vi "GetClassInfoDialog.vi"(0 "ClassWriterRefIn":refnum<class "ClassWriterNative.lvclass">, 1 "ClassItemRefIn":refnum<vi>, 5 "error in (no error)":errorcluster) -> (14 "ClassWriterRefOut":refnum<class "ClassWriterNative.lvclass">, 19 "error out":errorcluster)   [LabVIEW 2020, in "ClassWriterNative.lvclass"]
uses:
  <resource>/Framework/Providers/Open_GDS/ClassProviders/Provider_LvNativeClass/ClassWriterNative_class/ClassWriterNative.lvclass
  <resource>/Framework/Providers/Open_GDS/ClassProviders/Common/ScriptingFunctions/Scripting_ConnectorPanePatternType.ctl
  <resource>/Framework/Providers/Open_GDS/ClassProviders/Common/LvClass_class/GDSLvClass_PlugIn.ctl
  <resource>/Framework/Providers/Open_GDS/ClassProviders/Common/LvClass_class/GDSLvClass_PlugInTypes.ctl
  Instance           1 26Saved   GetClassInfoDialog .vi
panel:
  out "Connector Pane":T1 items=["4x4x4", "5x6x5", "6x8x6"]
  in  "_SaveChanges":bool
  in  "_ClassPlugIns":T2(array[cluster]) caption="PlugIns / Design Patterns"
  in  "_EditPlugIn":bool
  in  "_OK":bool
  out "_ClassDescription":string caption="Class description"
  out "_ClassTemplateVersion":string caption="Class Template Version"
  out "_ClassTemplateUsed":string caption="Class Template Used"
  out "_ClassProviderName":string caption="Class Provider Name"
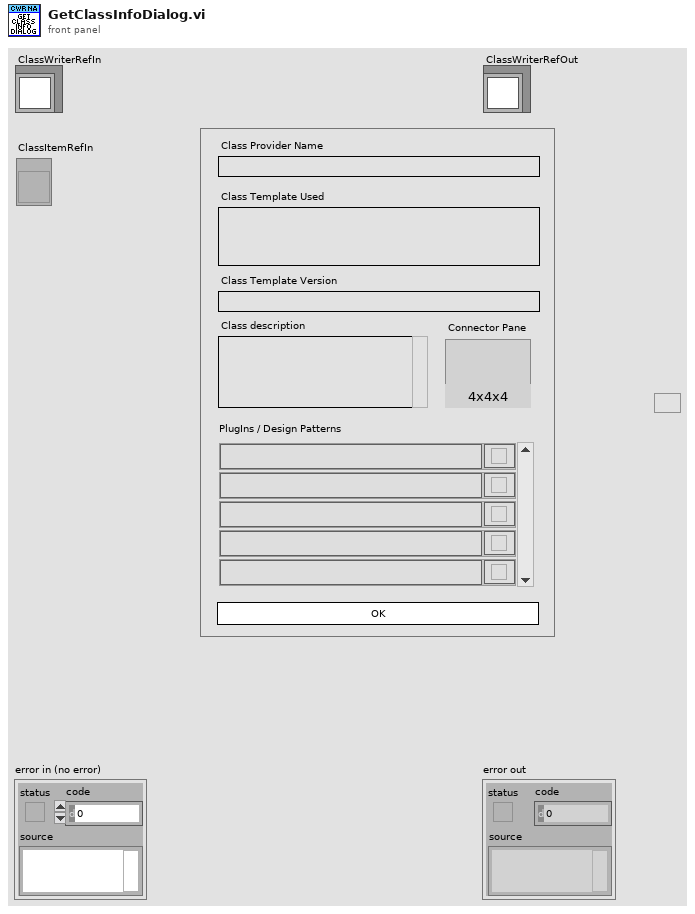
[diagram p1: front panel]
types:
  T1 = typedef "Scripting_ConnectorPanePatternType.ctl" = u16
  T2 = cluster{"_ClassPlugIn 2":string, "Remove":bool, "Block":bool}[]
  T3 = typedef "GDSLvClass_PlugIn.ctl" = cluster{"Type":T4, "ID":string, "Version":string, "Path":path, "Name":string, "Data":variant}
  T4 = typedef "GDSLvClass_PlugInTypes.ctl" = enum16{"DesignPattern", "MethodTypes"}
  T5 = cluster{"_ClassPlugIn 2":string, "_RemovePlugIn":bool, "Block":bool}
  T6 = typedef "GDSLvCLass_ClassSettingsType.ctl" = cluster{"ClassProviderName":string, "ClassTemplateUsed":string, "ClassTemplateVersion":string, "ClassDescription":string, "PlugIns":T3[], "ConnectorPanePattern":string}
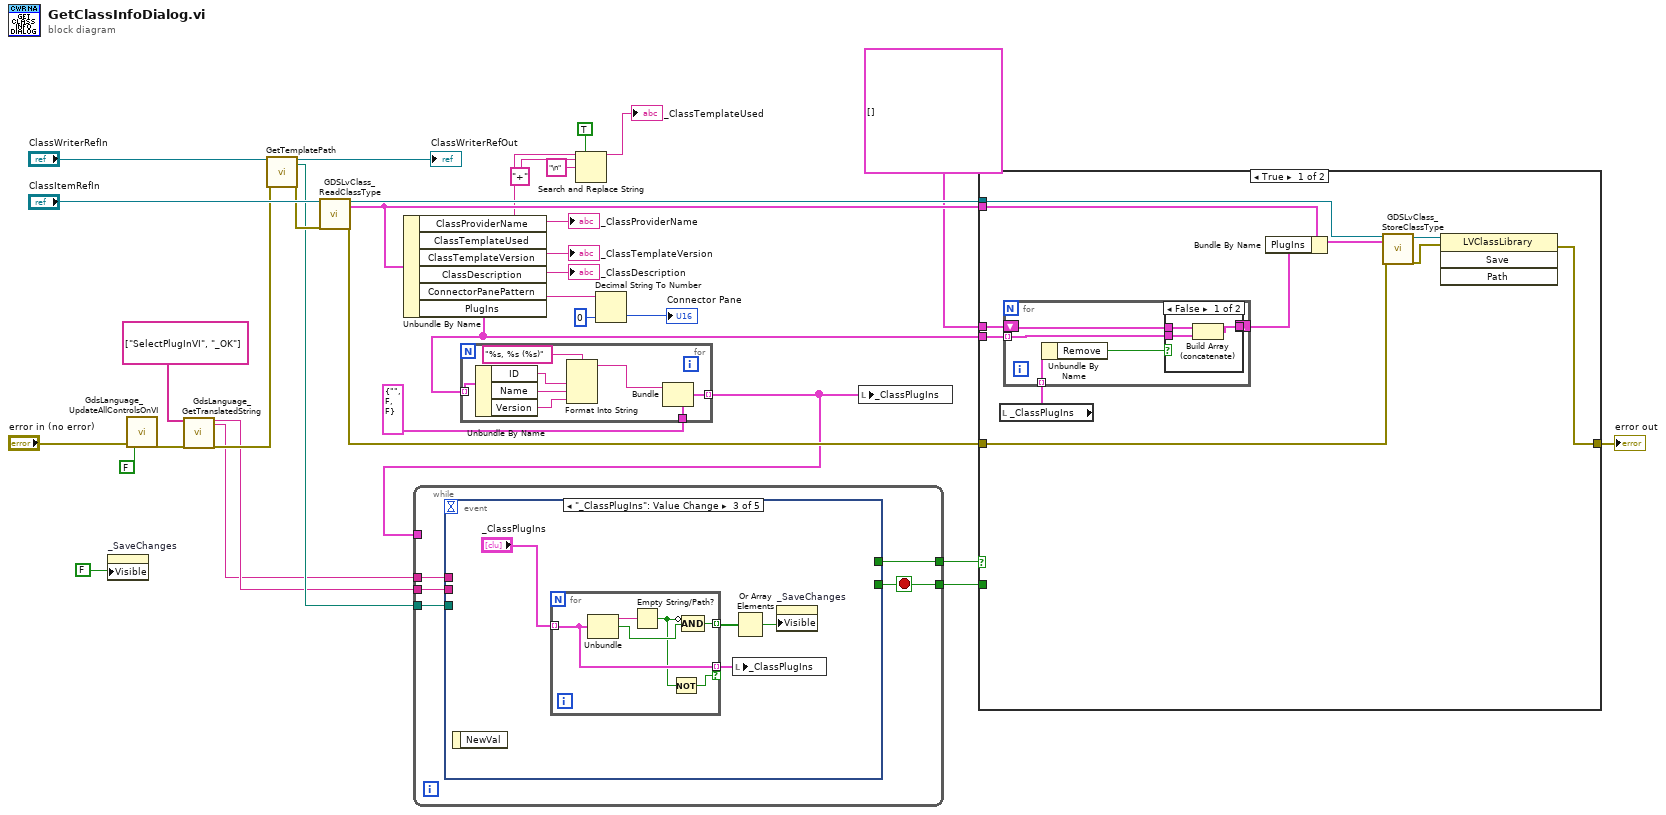
[diagram p0: block diagram]
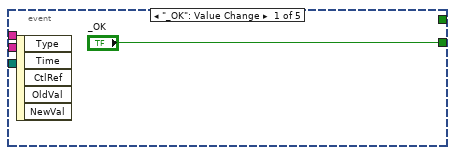
[diagram p4: hidden frame]
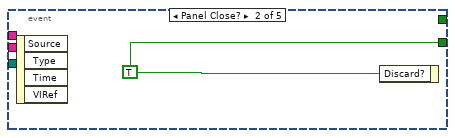
[diagram p5: hidden frame]
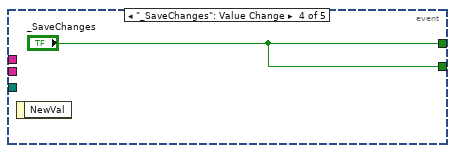
[diagram p6: hidden frame]
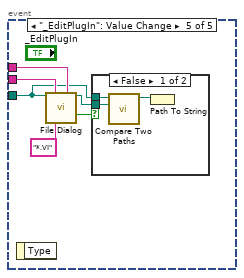
[diagram p7: hidden frame]
diagram:
  n1 = property on="_SaveChanges" class="Bool"("Visible"=FALSE) -> ()  [unwired: 2 in, 2 out]
  n2 = call <resource>:"GdsLanguage_UpdateAllControlsOnVI.vi"("error in (no error)"="error in (no error)", "CreateLanguageFile(Use this to create a languageFile)"=FALSE) -> ("error out"=w20:errorcluster)  [unwired: 16 in, 1 out]
  n3 = call <resource>:"GdsLanguage_GetTranslatedString.vi"("StringID(s)"=string[] ["SelectPlugInVI", "_OK"], "error in (no error)"=w20) -> ("FirstStringOut"=w17:string, "SecondStringOut"=w15:string, "error out"=w19:errorcluster)  [unwired: 14 in, 1 out]
  n4 = call-dynamic "GetTemplatePath.vi"("reference in"="ClassWriterRefIn", "error in (no error)"=w19) -> ("reference out"=→"ClassWriterRefOut":refnum<class "ClassWriterNative.lvclass">, "FolderPathOut"=w18:path, "error out"=w22:errorcluster)  [unwired: 13 in, 2 out]
  n5 = call <resource>:"GDSLvClass_ReadClassType.vi"("Class Refnum In"="ClassItemRefIn", "error in (no error)"=w22) -> ("Class Refnum Out"=w30:refnum<vi>, "ClassSettings"=w25:T6, "error out"=w29:errorcluster)  [unwired: 15 in]
  n6 = Unbundle By Name(w25) -> ("ClassProviderName"=→"_ClassProviderName":string, "ClassTemplateUsed"=w9:string, "ClassTemplateVersion"=→"_ClassTemplateVersion":string, "ClassDescription"=→"_ClassDescription":string, "ConnectorPanePattern"=w4:string, "PlugIns"=w12:T3[])
  n7 = for {
    tunnel: w12 -> [w40] mode=indexing
    tunnel: T5 {"_ClassPlugIn 2"="", "_RemovePlugIn"=FALSE, "Block"=FALSE} ("Cluster") -> [w42]
    tunnel: [w41] -> w1 mode=indexing
    n8 = Unbundle By Name(w40) -> ("ID"=w37:string, "Name"=w36:string, "Version"=w35:string)
    n9 = Format Into String(format string="%s, %s (%s)", w37, w36, w35) -> (resulting string=w38:string)  [unwired: 2 in, 1 out]
    n10 = Bundle(cluster=w42, "_ClassPlugIn 2"=w38) -> (w41:T5)  [unwired: 2 in]
  }
  n11 = while {
    tunnel: [w47] -> w24
    tunnel: w18 -> [w46]
    tunnel: w17 -> [w45]
    tunnel: w15 -> [w44]
    tunnel: [w43] -> w10
    tunnel: w1 -> [_]
    stop <- w47 stop-if-true
    n12 = event shown="[2] \"_ClassPlugIns\": Value Change" {
      selector: _ -> [_ _ _ _ _]
      dyn-events: _ -> [_ _ _ _ _]
      timeout: _ -> [_ _ _ _ _]
      tunnel: ["_OK" w49 _ "_SaveChanges" _] -> w47
      tunnel: w46 -> [_ _ _ _ w62]
      tunnel: w45 -> [_ _ _ _ w66]
      tunnel: w44 -> [_ _ _ _ w64]
      tunnel: [_ _ _ "_SaveChanges" _] -> w43
      event "_OK": Value Change {
        n13 = event-data() -> ()  [unwired: 1 in, 5 out]
      }
      event Panel Close? {
        w49 = TRUE ("Discard?")
        n14 = event-data() -> ()  [unwired: 1 in, 4 out]
        n15 = event-data("Discard?"=w49) -> ()  [unwired: 1 in, 1 out]
      }
      event "_ClassPlugIns": Value Change {
        n16 = event-data() -> ()  [unwired: 1 in, 1 out]
        n17 = for {
          tunnel: "_ClassPlugIns" -> [w57] mode=indexing
          tunnel: [w57] -> w52 mode=indexing if=w55
          tunnel: [w54] -> w51 mode=indexing
          n18 = Unbundle(w57) -> ("_ClassPlugIn 2"=w59:string, "Remove"=w58:bool)  [unwired: 1 out]
          n19 = Empty String/Path?(string/path=w59) -> (empty?=w56:bool)
          n20 = Not(x=w56) -> (.not. x?=w55:bool)
          n21 = Compound Arithmetic op=AND(invert w56, w58) -> (w54:bool)
        }
        n22 = local write "_ClassPlugIns"(w52) -> ()
        n23 = Or Array Elements(Boolean array=w51) -> (logical OR=w50:bool)
        n24 = property on="_SaveChanges" class="Bool"("Visible"=w50) -> ()  [unwired: 2 in, 2 out]
      }
      event "_SaveChanges": Value Change {
        n25 = event-data() -> ()  [unwired: 1 in, 1 out]
      }
      event "_EditPlugIn": Value Change {
        n26 = event-data() -> ()  [unwired: 1 in, 1 out]
        n27 = call "File Dialog"("start path"=w62, "prompt"=w66, "button label"=w64, "pattern (all files)"="*.VI") -> ("selected path"=w61:path, "cancelled"=w63:bool)  [unwired: 8 in, 2 out]
        n28 = case shown="False" w63 {
          tunnel: w62 -> [w69 _]
          tunnel: w61 -> [w68 _]
          frame False {
            n29 = call <vilib>:"Compare Two Paths.vi"("Path 2"=w68, "Path 1"=w69) -> ("Relative Path from 1 to 2"=w67:path)  [unwired: 6 in, 3 out]
            n30 = Path To String(path=w67) -> ()  [unwired: 1 out]
          }
          frame True {
          }
        }
      }
    }
  }
  n31 = Search and Replace String(replace all?=TRUE ("replace all? (F)"), input string=w9, search string="+", replace string="\n" ("replace string (\"\")")) -> (result string=→"_ClassTemplateUsed":string)  [unwired: 4 in, 3 out]
  n32 = Decimal String To Number(string=w4, default (0L)=u16 0 ("default (0 I32)")) -> (number=→"Connector Pane":u16)  [unwired: 1 in, 1 out]
  n33 = local write "_ClassPlugIns"(w1) -> ()
  n34 = case shown="True" w10 {
    tunnel: w30 -> [w80 _]
    tunnel: w29 -> [w79 w90]
    tunnel: [w78 w90] -> w28
    tunnel: w25 -> [w77 _]
    tunnel: w24 -> [_ _]
    tunnel: w12 -> [w75 _]
    tunnel: T3[] [] -> [w73 _]
    frame True {
      n35 = local read "_ClassPlugIns"() -> (w72:T2)
      n36 = for {
        tunnel: w75 -> [w83] mode=indexing
        shift-right: [w84] -> w74
        shift-left: w73 -> [w85]
        tunnel: w72 -> [w82] mode=indexing
        n37 = Unbundle By Name(w82) -> ("Remove"=w81:bool)
        n38 = case shown="False" w81 {
          tunnel: w85 -> [w88 w89]
          tunnel: w83 -> [w87 _]
          tunnel: [w86 w89] -> w84
          frame False {
            n39 = Build Array (concatenate)(w88, w87) -> (w86:T3[])
          }
          frame True {
          }
        }
      }
      n40 = Bundle By Name(cluster=w77, "PlugIns"=w74) -> (w76:T6)
      n41 = call <resource>:"GDSLvClass_StoreClassType.vi"("Class Refnum In"=w80, "ClassSettings"=w76, "error in (no error)"=w79) -> ("Class Refnum Out"=w71:refnum<vi>, "error out"=w70:errorcluster)  [unwired: 15 in]
      n42 = invoke class="LVClassLibrary" method="Save"(reference=w71, error in=w70) -> (error out=w78:errorcluster)  [unwired: 2 in, 3 out]
    }
    frame False {
    }
  }
  "error out" <- w28
